vi "vacuum_n.vi"(8 "error in (no error)":errorcluster, 10 "Vacuum Setting (0000)":i64 min=0 max=1000 step=1 format="%04.0f", 11 "Dispenser in":refnum<class "Dispenser.lvclass">) -> (0 "error out":errorcluster, 3 "Dispenser out":refnum<class "Dispenser.lvclass">)   [LabVIEW 2016]
uses:
  Classes/Controller/Dispenser/Dispenser Folder/Dispenser.lvclass
  Drivers/EFD Ultimus V/EFD Ultimus V.lvlib
panel:
  in  "VISA resource name":refnum<visa-resource-name>="COM1"
  in  "Vacuum Setting (0000) 2":i64 min=0 max=1000 step=1 format="%04.0f"
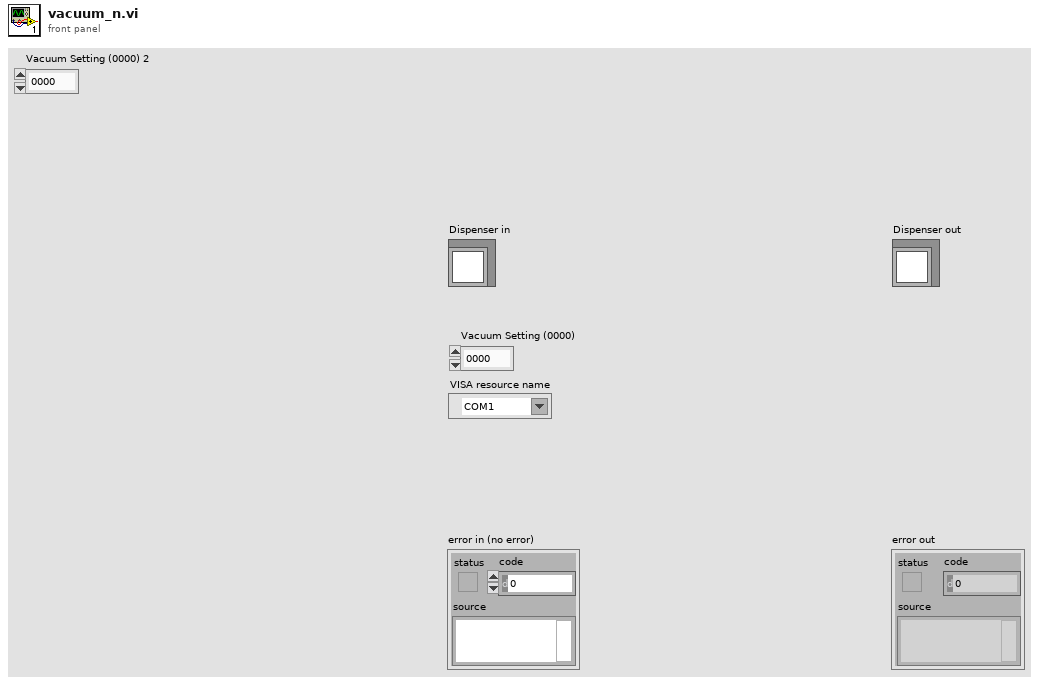
[diagram p1: front panel]
types:
  T1 = cluster{"Dispenser in":refnum<class "Dispenser.lvclass">, "VISA resource name":refnum<visa-resource-name>}
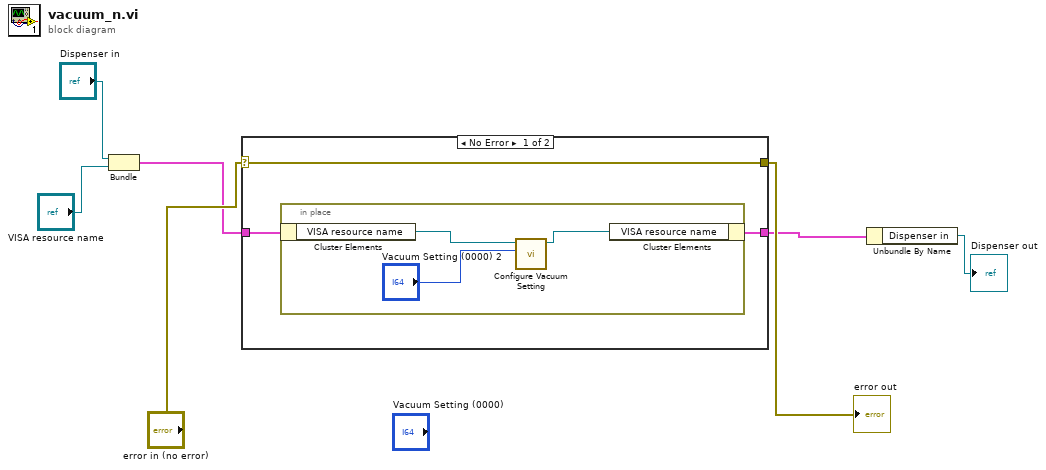
[diagram p0: block diagram]
diagram:
  n1 = Bundle("Dispenser in"="Dispenser in", "VISA resource name"="VISA resource name") -> (w3:T1)  [unwired: 1 in]
  n2 = case shown="No Error" "error in (no error)" {
    selector: "error in (no error)" -> [w10 w15]
    tunnel: w3 -> [w8 w14]
    tunnel: [w9 w14] -> w2
    tunnel: [w10 w15] -> w6
    frame No Error {
      n3 = in-place {
        n4 = in-place-cluster #1(w8) -> ("VISA resource name"=w13:refnum<visa-resource-name>)
        n5 = call "Configure Vacuum Setting.vi"("Vacuum Setting (0000)"="Vacuum Setting (0000) 2", "VISA resource name"=w13) -> ("VISA resource name out"=w12:refnum<visa-resource-name>)  [unwired: 8 in, 1 out]
        n6 = in-place-cluster #1("VISA resource name"=w12) -> (w9:T1)
      }
    }
    frame Error {
    }
  }
  "error out" <- w6
  n7 = Unbundle By Name(w2) -> ("Dispenser in"=→"Dispenser out":refnum<class "Dispenser.lvclass">)
